vi "多参数校准写入.vi"(8 "Error in":errorcluster caption="Error in (no error)", 9 "B":dbl caption="校准值B:", 10 "K":dbl caption="校准值K:", 11 "站号":u16(ring)=10 items=["氨氮"=3, "水温"=9, "pH值"=10, "溶解氧"=11, "电导率"=12, "浊度"=13, "叶绿素a"=14, "藻密度"=15, "蓝绿藻"=16, "氧化还原电位"=17, "溶解氧%"=18, "盐度"=19]) -> (0 "error out":errorcluster)   [LabVIEW 2016, in "斯坦道原位多参数.lvlib"]
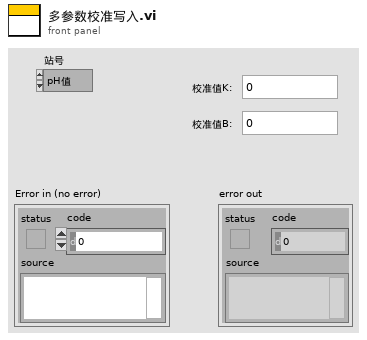
[diagram p1: front panel]
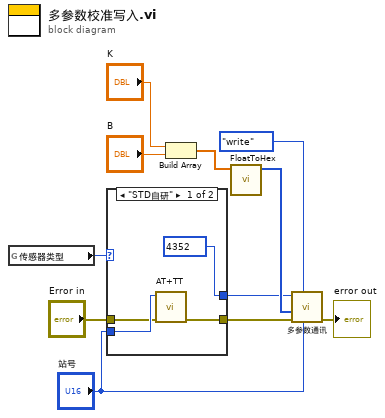
[diagram p0: block diagram]
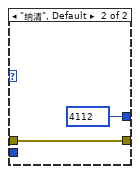
[diagram p2: hidden frame]
diagram:
  n1 = global read "多参数断电保存全局变量.vi" "传感器类型"() -> (w5:enum16{"STD自研", "纳清"})
  n2 = case shown="\"STD自研\"" w5 {
    tunnel: [u16 4352 ("starting address") u16 4112 ("starting address")] -> w4
    tunnel: "站号" -> [w14 _]
    tunnel: "Error in" -> [w13 w16]
    tunnel: [w12 w16] -> w1
    frame "STD自研" {
      n3 = call "AT+TT.vi"("错误输入（无错误）"=w13, "站号"=w14) -> ("错误输出"=w12:errorcluster)  [unwired: 9 in]
    }
    frame "纳清", Default {
    }
  }
  n4 = Build Array("K", "B") -> (w8:dbl[])
  n5 = call "FloatToHex.vi"("浮点数"=w8) -> ("DCBA整形输出"=w7:u16[])  [unwired: 10 in]
  n6 = call "多参数通讯.vi"("Slave ID"="站号", "STEP"=enum16{"open", "read", "write", "close"}."write", "Error in"=w1, "values"=w7, "starting address"=w4) -> ("error out"=→"error out":errorcluster)  [unwired: 4 in, 2 out]
